vi "PLL.vi"(8 "error in (no error)":errorcluster, 9 "sampling info":cluster{"Fs":dbl, "#s":dbl}, 10 "Lock-in parameters":T1, 11 "Refnum in":refnum<k21>) -> (0 "error out":errorcluster, 1 "photodiode":waveform(dbl), 2 "Cluster":cluster{"R":dbl, "Theta":dbl, "X":dbl, "Y":dbl}, 3 "Refnum out":refnum<k21>)   [LabVIEW 2015]
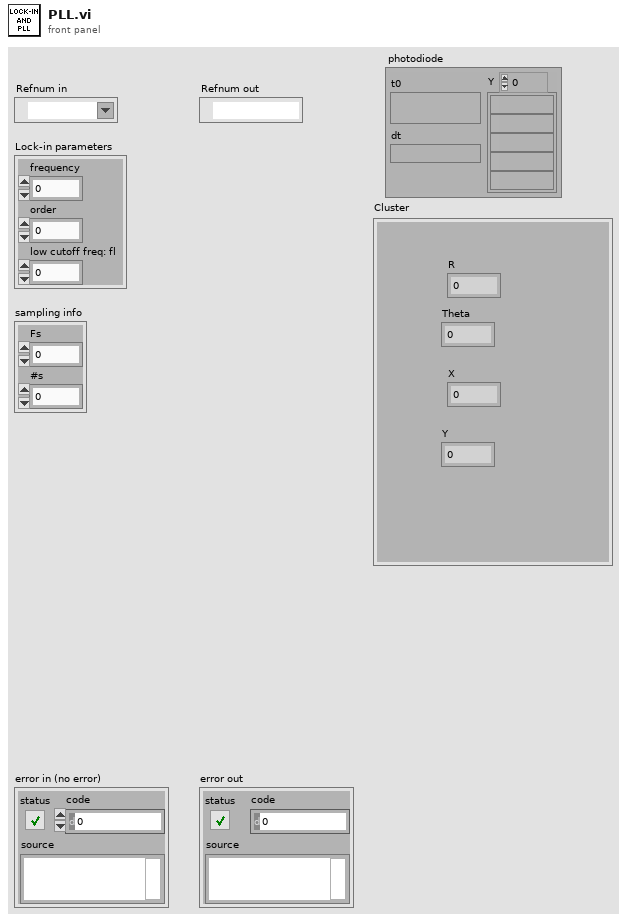
[diagram p1: front panel]
types:
  T1 = cluster{"frequency":dbl, "order":i32, "low cutoff freq: fl":dbl}
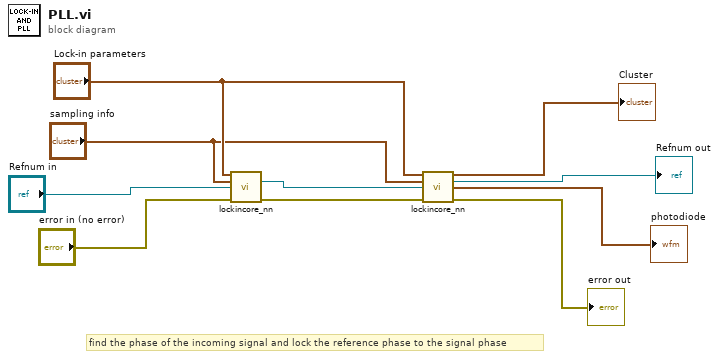
[diagram p0: block diagram]
diagram:
  # "find the phase of the incoming signal and lock the reference phase to the signal phase"
  n1 = call "lockincore_nn.vi"("Lock-in parameters"="Lock-in parameters", "sampling info"="sampling info", "task/channels in"="Refnum in", "error in (no error)"="error in (no error)") -> ("task out"=w8:refnum<k21>, "error out"=w5:errorcluster)  [unwired: 7 in, 3 out]
  n2 = call "lockincore_nn.vi"("Lock-in parameters"="Lock-in parameters", "sampling info"="sampling info", "task/channels in"=w8, "error in (no error)"=w5) -> ("Cluster"=→"Cluster":cluster{"R":dbl, "Theta":dbl, "X":dbl, "Y":dbl}, "task out"=→"Refnum out":refnum<k21>, "photodiode"=→"photodiode":waveform(dbl), "error out"=→"error out":errorcluster)  [unwired: 7 in, 1 out]
